vi "read dvr.vi"(8 "error in (no error)":errorcluster, 11 "NI-9237 in":refnum<class "NI-9237.lvclass">) -> (0 "error out":errorcluster, 2 "Numeric":dbl, 3 "NI-9237 out":refnum<class "NI-9237.lvclass">)   [LabVIEW 2025, in "Wheatstone Bridge.lvlib" / "NI-9237.lvclass"]
uses:
  NI-9237.lvclass
  NI-9237.lvclass/NI-9237.ctl
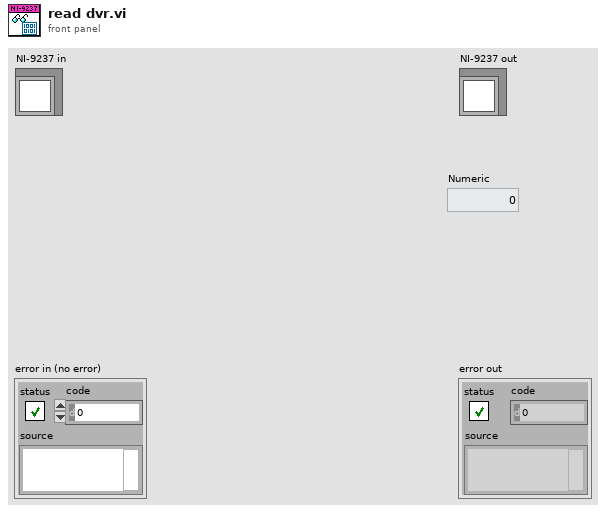
[diagram p1: front panel]
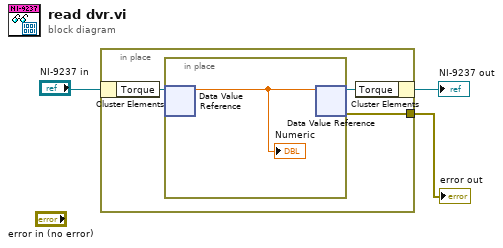
[diagram p0: block diagram]
diagram:
  n1 = in-place {
    in-place-border: [w4] -> w2
    n2 = in-place-cluster #1("NI-9237 in") -> ("Torque"=w6:refnum<data-value>)
    n3 = in-place {
      n4 = in-place-dvr #2(w6) -> (w7:dbl)  [unwired: 1 out]
      "Numeric" <- w7
      n5 = in-place-dvr #2(w7) -> (w5:refnum<data-value>, w4:errorcluster)
    }
    n6 = in-place-cluster #1("Torque"=w5) -> (→"NI-9237 out":refnum<class "NI-9237.lvclass">)
  }
  "error out" <- w2
